vi "testVi.vi"() -> ()   [LabVIEW 2011]
panel:
  in  "stop":bool
  # "THis is a test"
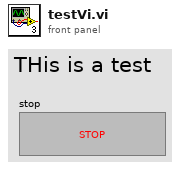
[diagram p1: front panel]
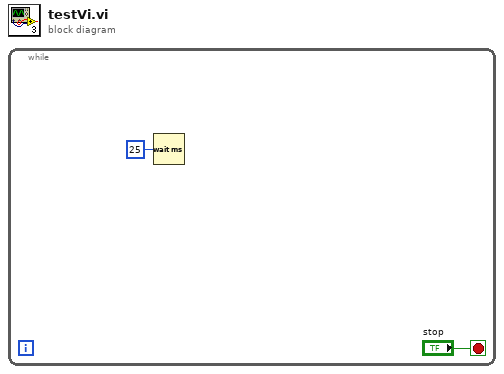
[diagram p0: block diagram]
diagram:
  n1 = while {
    stop <- "stop" stop-if-true
    n2 = Wait (ms)(milliseconds to wait=u32 25) -> ()  [unwired: 1 out]
  }
